vi "DM add burst.vi"(9 "mmWave data in":refnum<class "mmWave data.lvclass">, 10 "group":string, 11 "module loopdata in":T1) -> (1 "oldest":string, 2 "newest":string, 3 "module loopdata out":T1)   [LabVIEW 2019, in "DataManagment.lvlib"]
uses:
  DataManagment.lvlib
  module data.ctl
  SubVIs/mmWave data_class/mmWave data.lvclass
  DM signal group.ctl
  <vilib>/Utility/miscctls.llb/LVMapReplaceAction.ctl
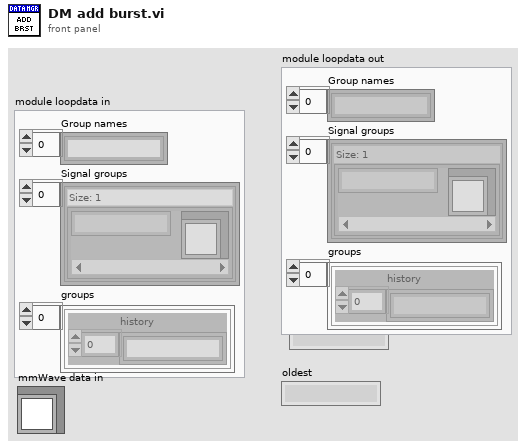
[diagram p1: front panel]
types:
  T1 = typedef "DataManagment.lvlib/module data.ctl" = cluster{"Group names":string[], "Signal groups":map{string, refnum<class "mmWave data.lvclass">}[], "groups":T2[]}
  T2 = typedef "DataManagment.lvlib/DM signal group.ctl" = cluster{"history":string[]}
  T3 = typedef "LVMapReplaceAction.ctl" = enum32{"Modify Entry only if found", "Add or Modify Entry", "Delete Entry"}
  T4 = map{string, refnum<class "mmWave data.lvclass">}[]
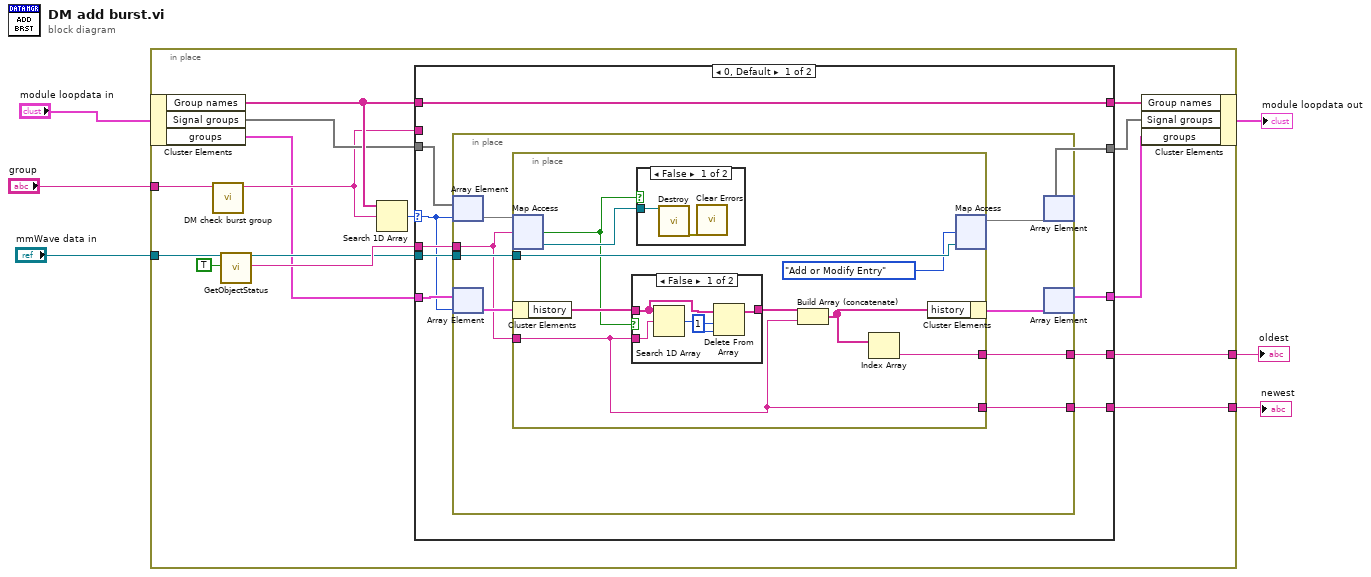
[diagram p0: block diagram]
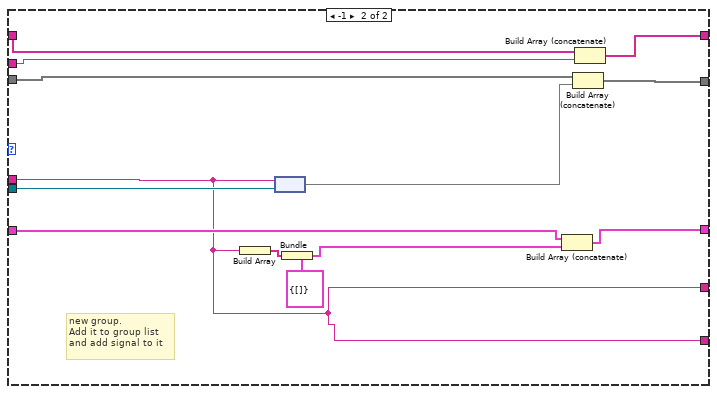
[diagram p4: hidden frame]
diagram:
  n1 = in-place {
    in-place-border: "group" -> [w12]
    in-place-border: "mmWave data in" -> [w17]
    in-place-border: [w8] -> w2
    in-place-border: [w7] -> w1
    n2 = in-place-cluster #1("module loopdata in") -> ("Group names"=w20:string[], "Signal groups"=w18:T4, "groups"=w10:T2[])
    n3 = call "DM check burst group.vi"("group"=w12) -> ("String"=w11:string)  [unwired: 10 in]
    n4 = call-dynamic "GetObjectStatus.vi"("reference in"=w17, "simple info (F)"=TRUE) -> ("reference out"=w13:refnum<class "mmWave data.lvclass">, "object name"=w14:string)  [unwired: 6 in, 10 out]
    n5 = Search 1D Array(1D array=w20, element=w11) -> (index of element=w21:i32)  [unwired: 1 in]
    n6 = case shown="0, Default" w21 {
      selector: w21 -> [w25 _]
      tunnel: w20 -> [w31 w69]
      tunnel: w11 -> [_ w63]
      tunnel: [w31 w68] -> w19
      tunnel: w18 -> [w30 w67]
      tunnel: w13 -> [w28 w66]
      tunnel: [w27 w64] -> w16
      tunnel: w14 -> [w29 w57]
      tunnel: w10 -> [w26 w62]
      tunnel: [w24 w58] -> w9
      tunnel: [w23 w57] -> w8
      tunnel: [w22 w57] -> w7
      frame 0, Default {
        n7 = in-place {
          in-place-border: w29 -> [w35]
          in-place-border: w28 -> [w38]
          in-place-border: [w33] -> w23
          in-place-border: [w32] -> w22
          n8 = in-place-array #2(w30, w25) -> (w39:map{string, refnum<class "mmWave data.lvclass">})
          n9 = in-place-array #3(w26, w25) -> (w36:T2)
          n10 = in-place {
            in-place-border: w38 -> [w48]
            in-place-border: w35 -> [w40]
            in-place-border: [w41] -> w33
            in-place-border: [w40] -> w32
            n11 = in-place-map #4(w39, w35) -> (w46:refnum<class "mmWave data.lvclass">, w44:bool)  [unwired: 1 in]
            n12 = in-place-cluster #5(w36) -> ("history"=w45:string[])
            n13 = case shown="False" w44 {
              tunnel: w45 -> [w51 w54]
              tunnel: w40 -> [w53 _]
              tunnel: [w50 w54] -> w43
              frame False {
                n14 = Search 1D Array(1D array=w51, element=w53) -> (index of element=w52:i32)  [unwired: 1 in]
                n15 = Delete From Array(array=w51, length=1, index=w52) -> (array with subset deleted=w50:string[])  [unwired: 1 out]
              }
              frame True {
              }
            }
            n16 = case shown="False" w44 {
              tunnel: w46 -> [w56 _]
              frame False {
                n17 = call-dynamic "Destroy.vi"("reference in"=w56) -> ("error out"=w55:errorcluster)  [unwired: 17 in, 1 out]
                n18 = call <vilib>:"Clear Errors.vi"("error in (no error)"=w55) -> ()  [unwired: 5 in, 2 out]
              }
              frame True {
              }
            }
            n19 = Build Array (concatenate)(w43, w40) -> (w42:string[])
            n20 = Index Array(array=w42) -> (element=w41:string)  [unwired: 1 in]
            n21 = in-place-cluster #5("history"=w42) -> (w34:T2)
            n22 = in-place-map #4(w48, LVMapReplaceAction."Add or Modify Entry" ("action")) -> (w37:map{string, refnum<class "mmWave data.lvclass">})  [unwired: 2 out]
          }
          n23 = in-place-array #2(w37) -> (w27:T4)  [unwired: 1 out]
          n24 = in-place-array #3(w34) -> (w24:T2[])  [unwired: 1 out]
        }
      }
      frame -1 {
        # "new group.\nAdd it to group list\nand add signal to it"
        n25 = Build Array(w57) -> (w61:string[])
        n26 = node(w57, w66) -> (w65:map{string, refnum<class "mmWave data.lvclass">})
        n27 = Bundle(cluster=T2 {"history"=[]} ("group"), "history"=w61) -> (w59:T2)
        n28 = Build Array (concatenate)(w62, w59) -> (w58:T2[])
        n29 = Build Array (concatenate)(w67, w65) -> (w64:T4)
        n30 = Build Array (concatenate)(w69, w63) -> (w68:string[])
      }
    }
    n31 = in-place-cluster #1("Group names"=w19, "Signal groups"=w16, "groups"=w9) -> (→"module loopdata out":T1)
  }
  "oldest" <- w2
  "newest" <- w1
